vi "run.vi"(8 "error in (no error)":errorcluster, 11 "TestCase in":refnum<class "TestCase.lvclass">) -> (0 "error out":errorcluster, 3 "TestCase out":refnum<class "TestCase.lvclass">)   [LabVIEW 2013, in "TestCase.lvclass"]
uses:
  TestCase.lvclass
panel:
  out "appended path":path
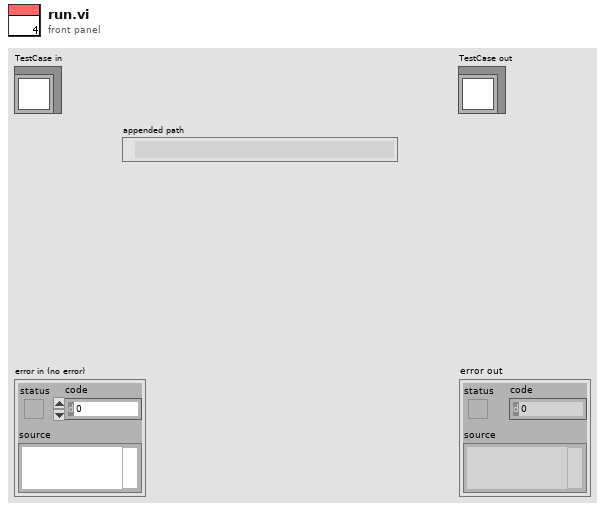
[diagram p1: front panel]
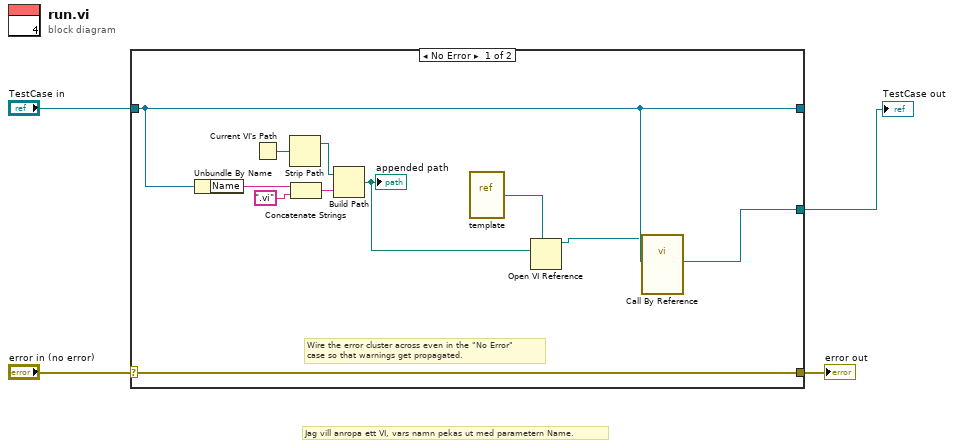
[diagram p0: block diagram]
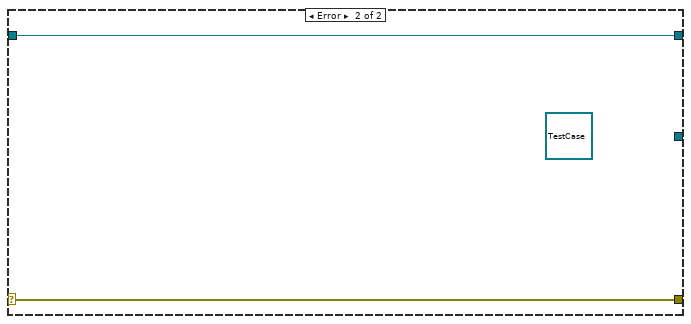
[diagram p2: hidden frame]
diagram:
  # "Jag vill anropa ett VI, vars namn pekas ut med parametern Name."
  n1 = case shown="No Error" "error in (no error)" {
    selector: "error in (no error)" -> [w10 w17]
    tunnel: [w10 w17] -> w3
    tunnel: [w8 w16] -> _
    tunnel: "TestCase in" -> [w8 w16]
    tunnel: [w5 _] -> w1
    frame No Error {
      # "Wire the error cluster across even in the \"No Error\"\ncase so that warnings get propagated."
      n2 = Unbundle By Name(w8) -> ("Name"=w12:string)
      n3 = Current VI's Path() -> (path=w15:path)
      n4 = Strip Path(path=w15) -> (stripped path=w14:path)  [unwired: 1 out]
      n5 = Concatenate Strings(w12, ".vi") -> (w11:string)
      n6 = Build Path(base path=w14, name or relative path=w11) -> (appended path=w9:path)
      "appended path" <- w9
      n7 = vi-ref "template.vi"() -> (w7:refnum<vi>)
      n8 = Open VI Reference(type specifier VI Refnum (for type only)=w7, vi path=w9) -> (vi reference=w6:refnum<vi>)  [unwired: 4 in, 1 out]
      n9 = call-by-ref "?"(reference=w6, "TestCase in"=w8) -> ("TestCase out"=w5:refnum<class "TestCase.lvclass">)  [unwired: 10 in, 3 out]
    }
    frame Error {
      (unwired) refnum<class "TestCase.lvclass"> refnum ("TestCase in")
    }
  }
  "error out" <- w3
  "TestCase out" <- w1
